vi "sine wave generator.vi"() -> ()   [LabVIEW 2009]
panel:
  out "Waveform Chart":dbl[](graph)
  in  "Numeric":dbl
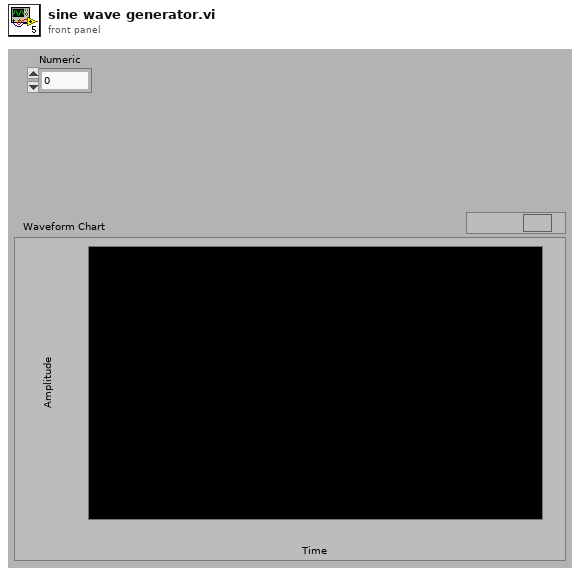
[diagram p1: front panel]
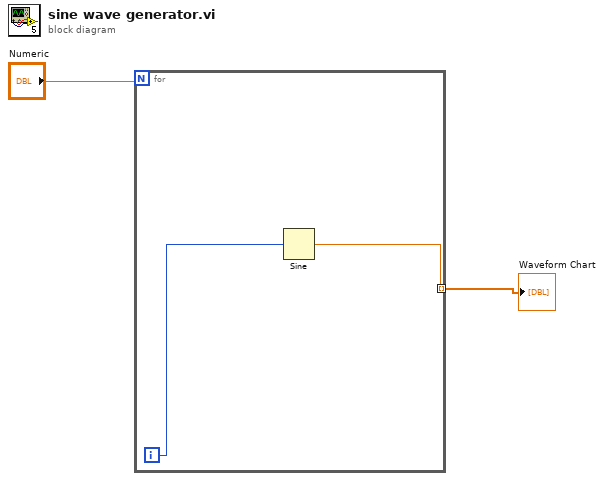
[diagram p0: block diagram]
diagram:
  n1 = for {
    N: "Numeric" -> [_]
    tunnel: [w3] -> w2 mode=indexing
    i -> [w4]
    n2 = Sine(x=w4) -> (sin(x)=w3:dbl)
  }
  "Waveform Chart" <- w2
